vi "Utility MODBUS RTU Receive Message.vi"(6 "Receive Message Type (0: By The Number Of Bytes)":u16(ring) items=["By The Number Of Bytes", "Copy Of The Sent Message"], 8 "error in (no error)":errorcluster, 9 "Sent Command (0)":u8, 10 "Length Of Sent MSG (0)":u8, 11 "VISA resource name":refnum<visa-resource-name>) -> (0 "error out":errorcluster, 1 "Read Buffer":u8[](array[numeric]), 3 "VISA resource name out":refnum<visa-resource-name>)   [LabVIEW 2014, in "Eurotherm 35xx Series.lvlib"]
doc: "VI - receive MODBUS RTU frame described by <B>Sent Command</B> control <LengthOfSentMSG> control (set out by MODBUS RTU Send Message.vi) and\nby selection <B>Receive Message Type</B>.\n\nThis VI is without message content decoding.\nSeparate usefull data message\nfrom the rest of the data frame and put it to the <B>read Buffer</B>.\nThe selector decode the frame by type of reading - \n\nAnswers can have 2 types:\n\n1. in answer frame is copy of the frame - is need to initialize on the input - <B>LengthOfSentMSG</B> and <B>Sent Command</B>, for right decoding\n\n2. answer frame consists information about length of main message in frame - The frame is divided automatically\n\n\nDescribed errors:\nBFFC09F1 - Bad in back protocol in Write Operation. Transmit Error.\nBFFC09F2 - Bad Received Message CRC\nBFFC09F3 - After WRITE: Error Statement, Error CRC\nBFFC09F4 - After WRITE: Register don't exist or is only for reading\nBFFC09F5 - After WRITE: data out of borders"
uses:
  <instrlib>/Eurotherm 35xx Series/Eurotherm 35xx Series.lvlib
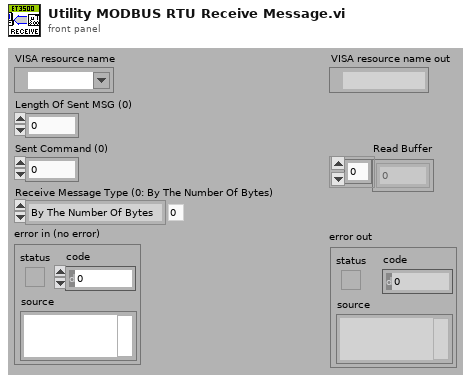
[diagram p1: front panel]
types:
  T1 = cluster{"unsigned byte array[0]":u8, "unsigned byte array[1]":u8}
  T2 = cluster{"status":bool, "code":i32, "VI Name":string}
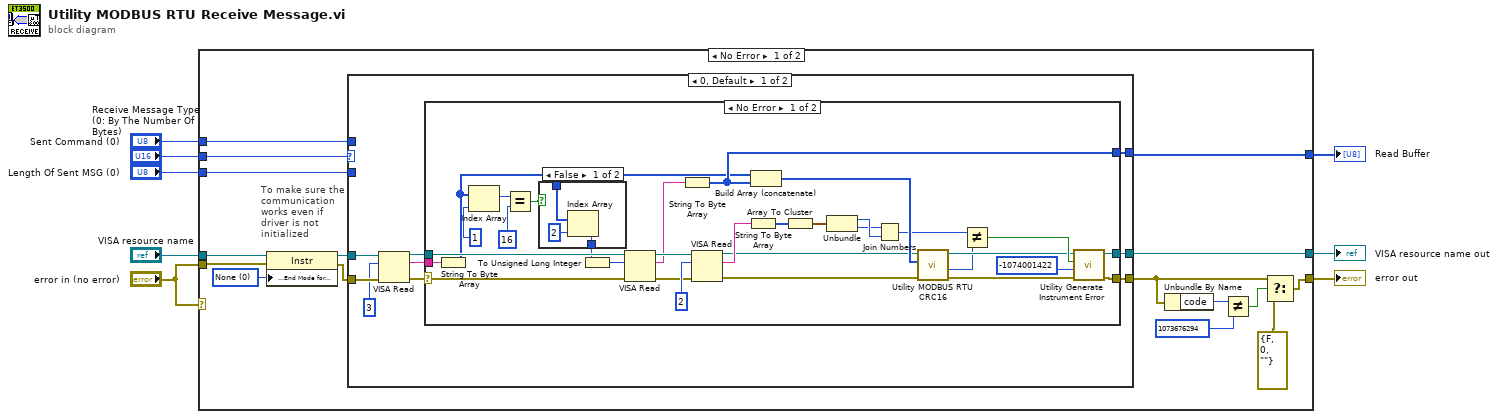
[diagram p0: block diagram]
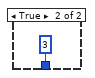
[diagram p2: hidden frame]
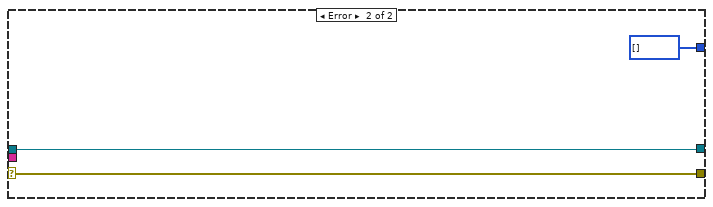
[diagram p3: hidden frame]
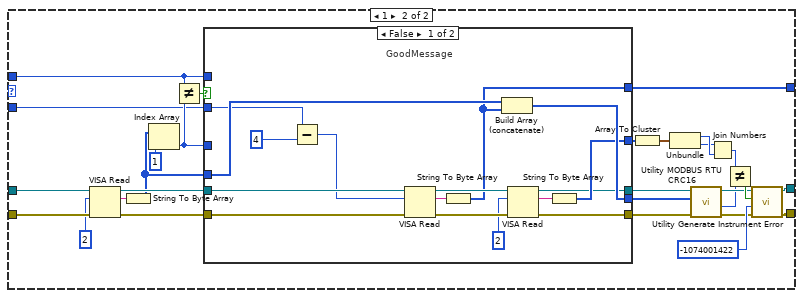
[diagram p4: hidden frame]
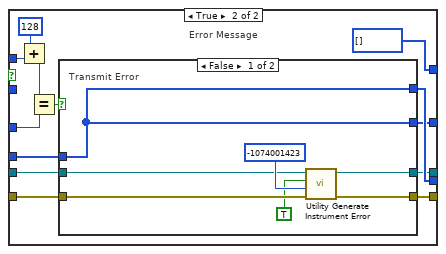
[diagram p5: hidden frame]
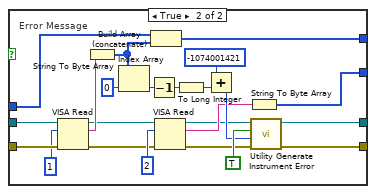
[diagram p6: hidden frame]
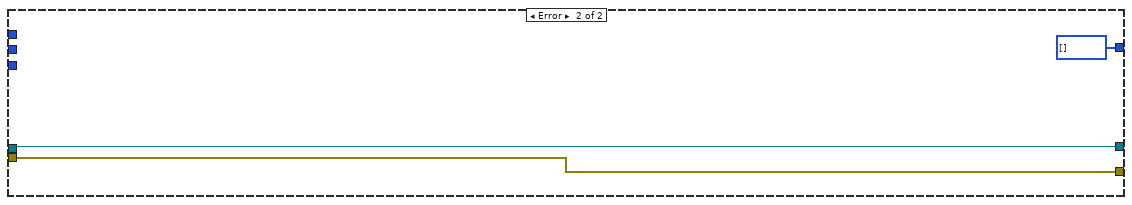
[diagram p7: hidden frame]
diagram:
  n1 = case shown="No Error" "error in (no error)" {
    tunnel: "error in (no error)" -> [w11 w160]
    tunnel: "Receive Message Type (0: By The Number Of Bytes)" -> [w24 _]
    tunnel: "VISA resource name" -> [w13 w159]
    tunnel: "Length Of Sent MSG (0)" -> [w23 _]
    tunnel: "Sent Command (0)" -> [w22 _]
    tunnel: [w21 u8[] [] ("unsigned byte array")] -> w4
    tunnel: [w15 w159] -> w2
    tunnel: [w14 w160] -> w1
    frame No Error {
      w9 = u16 0 items=["None", "LastBit", "TermChar"] ("Serial Settings:Serial End Mode for Reads")
      # "To make sure the\ncommunication \nworks even if\ndriver is not \ninitialized"
      n2 = property class="Instr"(reference=w13, error in=w11, "Serial Settings:End Mode for Reads"=w9) -> (reference out=w12:refnum<visa-resource-name>, error out=w10:errorcluster)
      n3 = case shown="0, Default" w24 {
        tunnel: [w28 w96] -> w20
        tunnel: w10 -> [w33 w98]
        tunnel: w12 -> [w31 w99]
        tunnel: [w26 w80] -> w15
        tunnel: [w25 w81] -> w21
        tunnel: w23 -> [_ w72]
        tunnel: w22 -> [_ w84]
        frame 0, Default {
          n4 = VISA Read(VISA resource name=w31, byte count=u32 3 ("byte count (0)"), error in (no error)=w33) -> (VISA resource name out=w27:refnum<visa-resource-name>, read buffer=w30:string, error out=w29:errorcluster)  [unwired: 1 out]
          n5 = case shown="No Error" w29 {
            selector: w29 -> [w63 w71]
            tunnel: w30 -> [w64 _]
            tunnel: [w51 w71] -> w28
            tunnel: w27 -> [w62 w70]
            tunnel: [w47 u8[] [] ("unsigned byte array")] -> w25
            tunnel: [w43 w70] -> w26
            frame No Error {
              n6 = String To Byte Array(string=w64) -> (unsigned byte array=w35:u8[])
              n7 = Index Array(array=w35, index=1) -> (element=w37:u8)
              n8 = Equal?(x=w37, y=u8 16 ("x")) -> (x = y?=w36:bool)
              n9 = case shown="False" w36 {
                tunnel: [w66 u8 3] -> w34
                tunnel: w35 -> [w65 _]
                frame False {
                  n10 = Index Array(array=w65, index=2) -> (element=w66:u8)
                }
                frame True {
                }
              }
              n11 = To Unsigned Long Integer(number=w34) -> (unsigned 32bit integer=w40:u32)
              n12 = VISA Read(VISA resource name=w62, byte count=w40, error in (no error)=w63) -> (VISA resource name out=w59:refnum<visa-resource-name>, read buffer=w57:string, error out=w58:errorcluster)  [unwired: 1 out]
              n13 = String To Byte Array(string=w57) -> (unsigned byte array=w47:u8[])
              n14 = VISA Read(VISA resource name=w59, byte count=u32 2 ("byte count (0)"), error in (no error)=w58) -> (VISA resource name out=w45:refnum<visa-resource-name>, read buffer=w61:string, error out=w56:errorcluster)  [unwired: 1 out]
              n15 = String To Byte Array(string=w61) -> (unsigned byte array=w55:u8[])
              n16 = Build Array (concatenate)(w35, w47) -> (w46:u8[])
              n17 = Array To Cluster(array=w55) -> (cluster=w54:T1)
              n18 = Unbundle(w54) -> ("unsigned byte array[0]"=w53:u8, "unsigned byte array[1]"=w52:u8)
              n19 = Join Numbers(hi=w52, lo=w53) -> ((hi.lo)=w42:u16)
              n20 = call <instrlib>:"Utility MODBUS RTU CRC16.vi"("error in (no error)"=w56, "Message (empty array)"=w46, "VISA resource name"=w45) -> ("error out"=w49:errorcluster, "CRC"=w41:u16, "VISA resource name out"=w44:refnum<visa-resource-name>)  [unwired: 5 in, 1 out]
              n21 = Not Equal?(x=w42, y=w41) -> (x != y?=w50:bool)
              n22 = call <instrlib>:"Utility Generate Instrument Error.vi"("error in (no error)"=w49, "Code (0)"=-1074001422, "Status (F: Off)"=w50, "VISA resource name"=w44) -> ("error out"=w51:errorcluster, "VISA resource name out"=w43:refnum<visa-resource-name>)  [unwired: 6 in]
            }
            frame Error {
            }
          }
        }
        frame 1 {
          n23 = VISA Read(VISA resource name=w99, byte count=u32 2 ("byte count (0)"), error in (no error)=w98) -> (VISA resource name out=w97:refnum<visa-resource-name>, read buffer=w73:string, error out=w88:errorcluster)  [unwired: 1 out]
          n24 = String To Byte Array(string=w73) -> (unsigned byte array=w82:u8[])
          n25 = Index Array(array=w82, index=1) -> (element=w85:u8)
          n26 = Not Equal?(x=w84, y=w85) -> (x != y?=w86:bool)
          n27 = case shown="False" w86 {
            tunnel: w97 -> [w114 w128]
            tunnel: [w105 w119] -> w91
            tunnel: [w111 w121] -> w79
            tunnel: w88 -> [w115 w127]
            tunnel: w85 -> [_ w126]
            tunnel: w84 -> [_ w117]
            tunnel: [w107 w123] -> w83
            tunnel: w82 -> [w113 w122]
            tunnel: [w104 w120] -> w78
            tunnel: [w103 u8[] [] ("unsigned byte array")] -> w81
            tunnel: w72 -> [w102 _]
            frame False {
              # "GoodMessage"
              n28 = Subtract(x=w102, y=u8 4) -> (x-y=w101:u8)
              n29 = VISA Read(VISA resource name=w114, byte count=w101, error in (no error)=w115) -> (VISA resource name out=w109:refnum<visa-resource-name>, read buffer=w112:string, error out=w110:errorcluster)  [unwired: 1 out]
              n30 = String To Byte Array(string=w112) -> (unsigned byte array=w103:u8[])
              n31 = Build Array (concatenate)(w113, w103) -> (w111:u8[])
              n32 = VISA Read(VISA resource name=w109, byte count=u32 2 ("byte count (0)"), error in (no error)=w110) -> (VISA resource name out=w104:refnum<visa-resource-name>, read buffer=w106:string, error out=w107:errorcluster)  [unwired: 1 out]
              n33 = String To Byte Array(string=w106) -> (unsigned byte array=w105:u8[])
            }
            frame True {
              # "Error Message"
              n34 = Add(x=u8 128 ("y"), y=w117) -> (x+y=w125:u8)
              n35 = Equal?(x=w125, y=w126) -> (x = y?=w124:bool)
              n36 = case shown="False" w124 {
                tunnel: w128 -> [w130 w158]
                tunnel: w127 -> [w134 w157]
                tunnel: [w133 w136] -> w123
                tunnel: w122 -> [w131 w146]
                tunnel: [w131 w145] -> w121
                tunnel: [w129 w137] -> w120
                tunnel: [w131 w142] -> w119
                frame False {
                  # "Transmit Error"
                  n37 = call <instrlib>:"Utility Generate Instrument Error.vi"("error in (no error)"=w134, "Code (0)"=-1074001423, "Status (F: Off)"=TRUE ("status"), "VISA resource name"=w130) -> ("error out"=w133:errorcluster, "VISA resource name out"=w129:refnum<visa-resource-name>)  [unwired: 6 in]
                }
                frame True {
                  # "Error Message"
                  n38 = VISA Read(VISA resource name=w158, byte count=u32 1 ("byte count (0)"), error in (no error)=w157) -> (VISA resource name out=w141:refnum<visa-resource-name>, read buffer=w154:string, error out=w140:errorcluster)  [unwired: 1 out]
                  n39 = String To Byte Array(string=w154) -> (unsigned byte array=w153:u8[])
                  n40 = Index Array(array=w153, index=0) -> (element=w151:u8)
                  n41 = Decrement(x=w151) -> (x-1=w148:u8)
                  n42 = Build Array (concatenate)(w146, w153) -> (w145:u8[])
                  n43 = VISA Read(VISA resource name=w141, byte count=u32 2 ("byte count (0)"), error in (no error)=w140) -> (VISA resource name out=w138:refnum<visa-resource-name>, read buffer=w143:string, error out=w139:errorcluster)  [unwired: 1 out]
                  n44 = To Long Integer(number=w148) -> (32bit integer=w147:i32)
                  n45 = Add(x=-1074001421, y=w147) -> (x+y=w149:i32)
                  n46 = String To Byte Array(string=w143) -> (unsigned byte array=w142:u8[])
                  n47 = call <instrlib>:"Utility Generate Instrument Error.vi"("error in (no error)"=w139, "Code (0)"=w149, "Status (F: Off)"=TRUE ("status"), "VISA resource name"=w138) -> ("error out"=w136:errorcluster, "VISA resource name out"=w137:refnum<visa-resource-name>)  [unwired: 6 in]
                }
              }
            }
          }
          n48 = Array To Cluster(array=w91) -> (cluster=w94:T1)
          n49 = Unbundle(w94) -> ("unsigned byte array[0]"=w93:u8, "unsigned byte array[1]"=w92:u8)
          n50 = call <instrlib>:"Utility MODBUS RTU CRC16.vi"("error in (no error)"=w83, "Message (empty array)"=w79, "VISA resource name"=w78) -> ("error out"=w89:errorcluster, "CRC"=w76:u16, "VISA resource name out"=w77:refnum<visa-resource-name>)  [unwired: 5 in, 1 out]
          n51 = Join Numbers(hi=w92, lo=w93) -> ((hi.lo)=w75:u16)
          n52 = Not Equal?(x=w75, y=w76) -> (x != y?=w90:bool)
          n53 = call <instrlib>:"Utility Generate Instrument Error.vi"("error in (no error)"=w89, "Code (0)"=-1074001422, "Status (F: Off)"=w90, "VISA resource name"=w77) -> ("error out"=w96:errorcluster, "VISA resource name out"=w80:refnum<visa-resource-name>)  [unwired: 6 in]
        }
      }
      n54 = Unbundle By Name(w20) -> ("code"=w19:i32)
      n55 = Not Equal?(x=w19, y=1073676294) -> (x != y?=w17:bool)
      n56 = Select(t=w20, s=w17, f=cluster{bool, i32, "VI Name":string} {FALSE, 0, "VI Name"=""}) -> (s? t:f=w14:T2)
    }
    frame Error {
    }
  }
  "error out" <- w1
  "VISA resource name out" <- w2
  "Read Buffer" <- w4
